vi "mod_Generate Fractional Resampler FIR Coefficients v2.vi"() -> (0 "effective filter length":i32, 1 "interpolation factor":i32, 2 "extended length":i32, 3 "polyphase filter":dbl[](array[numeric]))   [LabVIEW 2020, in "niAMT.lvlib"]
uses:
  <vilib>/addons/Modulation/niAMT.lvlib
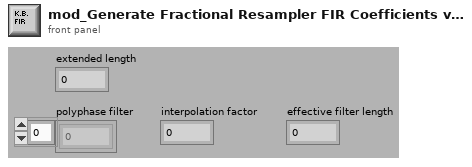
[diagram p1: front panel]
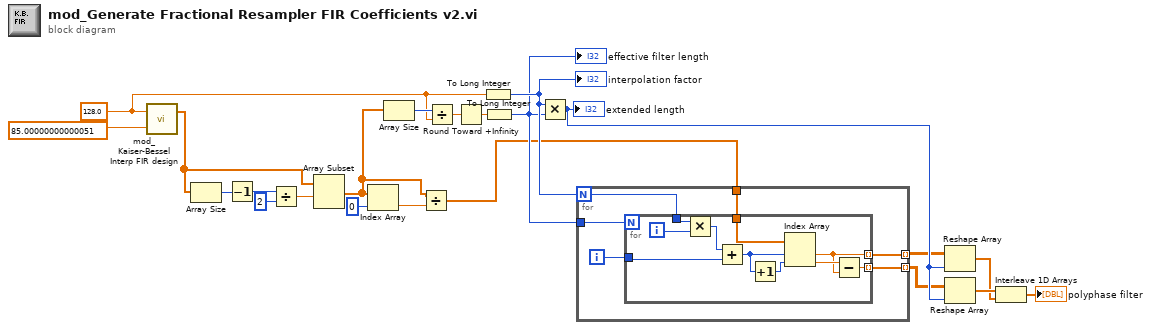
[diagram p0: block diagram]
diagram:
  w18 = 128.0 ("interpolation factor")
  n1 = call <vilib>:"mod_Kaiser-Bessel Interp FIR design.vi"("Stop Attenuation"=85.00000000000051, "interpolation factor"=w18) -> ("h"=w11:dbl[])  [unwired: 1 out]
  n2 = Array Size(array=w11) -> (size(s)=w15:i32)
  n3 = Decrement(x=w15) -> (x-1=w14:i32)
  n4 = Divide(x=w14, y=2) -> (x/y=w12:dbl)
  n5 = Array Subset(array=w11, index=w12) -> (w2:dbl[])  [unwired: 1 in]
  n6 = Index Array(array=w2, index=0) -> (element=w3:dbl)
  n7 = Array Size(array=w2) -> (size(s)=w21:i32)
  n8 = Divide(x=w2, y=w3) -> (x/y=w1:dbl[])
  n9 = Divide(x=w21, y=w18) -> (x/y=w20:dbl)
  n10 = Round Toward +Infinity(x=w20) -> (ceil(x): smallest int >= x=w19:dbl)
  n11 = To Long Integer(number=w18) -> (32bit integer=w17:i32)
  "interpolation factor" <- w17
  n12 = To Long Integer(number=w19) -> (32bit integer=w16:i32)
  "effective filter length" <- w16
  n13 = Multiply(x=w17, y=w16) -> (x*y=w10:i32)
  "extended length" <- w10
  n14 = for {
    N: w17 -> [w27]
    tunnel: w1 -> [w26]
    tunnel: [w25] -> w9 mode=indexing
    tunnel: w16 -> [w24]
    tunnel: [w23] -> w8 mode=indexing
    i -> [w28]
    n15 = for {
      N: w24 -> [_]
      tunnel: w28 -> [w35]
      tunnel: w27 -> [w37]
      tunnel: w26 -> [w34]
      tunnel: [w30] -> w25 mode=indexing
      tunnel: [w29] -> w23 mode=indexing
      i -> [w38]
      n16 = Multiply(x=w37, y=w38) -> (x*y=w36:i32)
      n17 = Add(x=w36, y=w35) -> (x+y=w32:i32)
      n18 = Increment(x=w32) -> (x+1=w33:i32)
      n19 = Index Array(array=w34, index #1=w32, index #2=w33) -> (element #1=w30:dbl, element #2=w31:dbl)
      n20 = Subtract(x=w31, y=w30) -> (x-y=w29:dbl)
    }
  }
  n21 = Reshape Array(w9, w10) -> (w6:dbl[])
  n22 = Reshape Array(w8, w10) -> (w7:dbl[])
  n23 = Interleave 1D Arrays(w7, w6) -> (→"polyphase filter":dbl[])
